vi "BoldTag.vi"(8 "error in (no error)":errorcluster, 11 "Bold in":refnum<class "Bold.lvclass">) -> (0 "error out":errorcluster, 2 "BoldTag":string, 3 "Bold out":refnum<class "Bold.lvclass">)   [LabVIEW 2021, in "LvMarkdown.lvlib" / "Bold.lvclass"]
uses:
  Bold.lvclass
  Bold.lvclass/Bold.ctl
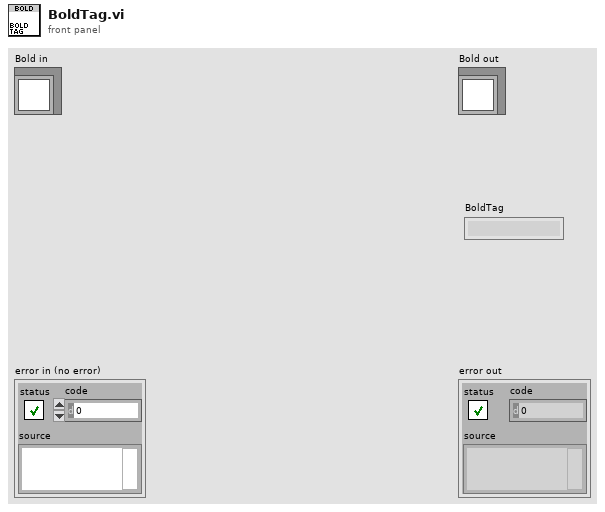
[diagram p1: front panel]
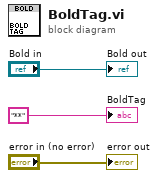
[diagram p0: block diagram]
diagram:
  "error out" <- "error in (no error)"
  "Bold out" <- "Bold in"
  "BoldTag" <- "**" ("BoldTag")
